vi "Value Prompt Async.vi"(7 "VolatusAPI":refnum<class "VolatusAPI.lvclass">, 11 "DblPopupControl in":refnum<class "DblPopupControl.lvclass">) -> ()   [LabVIEW 2020, in "VolatusGUIElements.lvlib" / "DblPopupControl.lvclass"]
uses:
  DblPopupControl.lvclass
  C:/dev/lv20CE/relink/lv-volatus/VolatusGUI/GUI Element/GUI Element.lvclass
  Volatus/VolatusAPI/VolatusAPI.lvclass
  DblPopupControl.lvclass/DblPopupControl.ctl
  lv-vecto/Vecto/Channel DBL/Channel DBL.lvclass/Channel DBL.ctl
  VolatusGUI/GUI Element/GUI Element.lvclass/GUI Element.ctl
  lv-vecto/Vecto/Group DBL/Value by Index.vi
  Volatus/VolatusAPI/Report Event.vi
  lv-vecto/Vecto/Channel DBL/Channel DBL.lvclass
  VolatusGUI/GUI Element/GUI Element.lvclass
  C:/dev/lv20CE/relink/lv-volatus/VolatusGUIElements/DblPopupControl/DblPopupControl.lvclass
  C:/dev/lv20CE/relink/lv-volatus/VolatusGUI/OnMouseDown/OnMouseDown.lvclass
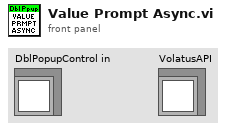
[diagram p1: front panel]
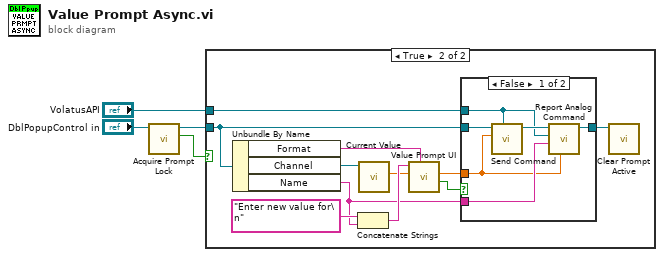
[diagram p0: block diagram]
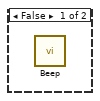
[diagram p2: hidden frame]
diagram:
  n1 = call "Acquire Prompt Lock.vi"("GUI Element in"="DblPopupControl in") -> ("Acquired"=w1:bool, "GUI Element out"=w2:refnum<class "DblPopupControl.lvclass">)  [unwired: 8 in, 1 out]
  n2 = case shown="True" w1 {
    tunnel: "VolatusAPI" -> [_ w10]
    tunnel: w2 -> [_ w5]
    frame False {
      n3 = call <vilib>:"Beep.vi"() -> ()  [unwired: 12 in]
    }
    frame True {
      n4 = Unbundle By Name(w5) -> ("Format"=w15:string, "Channel"=w9:refnum<class "Channel DBL.lvclass">, "Name"=w7:string)
      n5 = Concatenate Strings("Enter new value for\n", w7) -> (w13:string)
      n6 = call "Current Value.vi"("Channel in"=w9) -> ("Scaled"=w8:dbl)  [unwired: 6 in, 4 out]
      n7 = call "Value Prompt UI.vi"("Display Format"=w15, "Default"=w8, "Prompt"=w13) -> ("Cancelled"=w12:bool, "New Value"=w11:dbl)  [unwired: 7 in]
      n8 = case shown="False" w12 {
        tunnel: w11 -> [w17 _]
        tunnel: w5 -> [w21 w22]
        tunnel: w10 -> [w19 _]
        tunnel: w7 -> [w18 _]
        tunnel: [w16 w22] -> w6
        frame False {
          n9 = call "Send Command.vi"("VolatusAPI"=w19, "Value"=w17, "DblPopupControl in"=w21) -> ("DblPopupControl out"=w20:refnum<class "DblPopupControl.lvclass">)  [unwired: 7 in, 1 out]
          n10 = call "Report Analog Command.vi"("Value"=w17, "Name"=w18, "VolatusAPI in"=w19, "GUI Element in"=w20) -> ("GUI Element out"=w16:refnum<class "DblPopupControl.lvclass">)  [unwired: 6 in, 1 out]
        }
        frame True {
        }
      }
      n11 = call "Clear Prompt Active.vi"("GUI Element in"=w6) -> ()  [unwired: 9 in, 2 out]
    }
  }
